vi "Params[LSTM[Gate]].vi"(1 "N":u64=2, 4 "M":u64=2) -> (18 "params[LSTM[gate]]":T2)   [LabVIEW 2014]
uses:
  <vilib>/Analysis/Matrix/Datatypes/RealMatrix.ctl
  <vilib>/Analysis/Matrix/NI_Matrix.lvlib
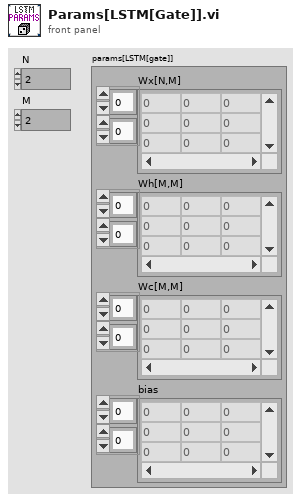
[diagram p1: front panel]
types:
  T1 = typedef "NI_Matrix.lvlib/RealMatrix.ctl" = dbl[][]
  T2 = cluster{"Wx[N,M]":T1, "Wh[M,M]":T1, "Wc[M,M]":T1, "bias":T1}
  T3 = cluster{"Normal Matrix":T1, "Normal Matrix":T1, "Normal Matrix":T1, "Normal Matrix":T1}
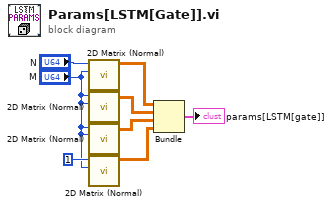
[diagram p0: block diagram]
diagram:
  n1 = call "2D Matrix (Normal).vi"("nRows"="M", "nCols"="N") -> ("Normal Matrix"=w7:T1)  [unwired: 9 in]
  n2 = call "2D Matrix (Normal).vi"("nRows"="M", "nCols"="M") -> ("Normal Matrix"=w6:T1)  [unwired: 9 in]
  n3 = call "2D Matrix (Normal).vi"("nRows"="M", "nCols"="M") -> ("Normal Matrix"=w5:T1)  [unwired: 9 in]
  n4 = call "2D Matrix (Normal).vi"("nRows"="M", "nCols"=1) -> ("Normal Matrix"=w4:T1)  [unwired: 9 in]
  n5 = Bundle("Normal Matrix"=w7, "Normal Matrix"=w6, "Normal Matrix"=w5, "Normal Matrix"=w4) -> (→"params[LSTM[gate]]":T3)  [unwired: 1 in]
